vi "Formula Node.vi"() -> ()   [LabVIEW 2022 SP3]
panel:
  out "x":dbl
  in  "C":dbl
  in  "B":dbl
  in  "A":dbl
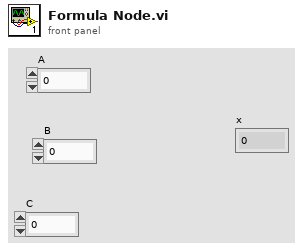
[diagram p1: front panel]
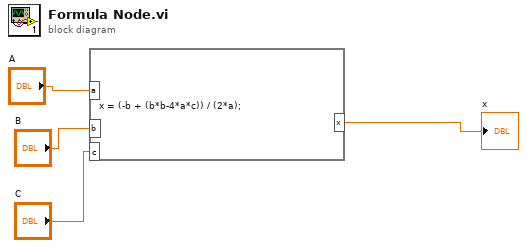
[diagram p0: block diagram]
diagram:
  n1 = formula code="x = (-b + (b*b-4*a*c)) / (2*a);"("a"="A", "b"="B", "c"="C") -> ("x"=→"x":dbl)
